vi "Deflate IWT Coeff.vi"(8 "error in (no error)":errorcluster, 11 "IWT coef":T1(array[cluster])) -> (0 "error out":errorcluster, 2 "Length":i32=1051714, 3 "data string":string)   [LabVIEW 2023]
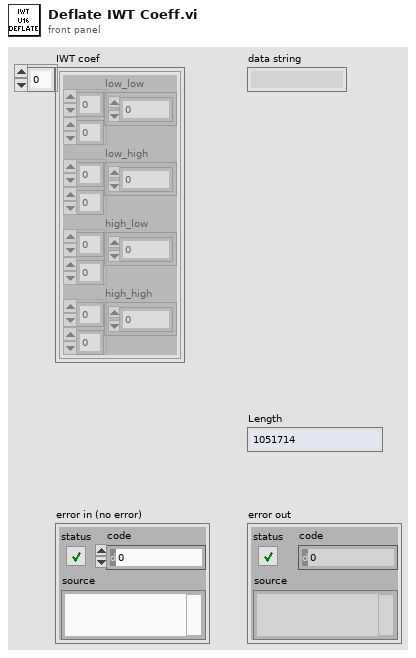
[diagram p1: front panel]
types:
  T1 = cluster{"low_low":i32[][], "low_high":i32[][], "high_low":i32[][], "high_high":i32[][]}[]
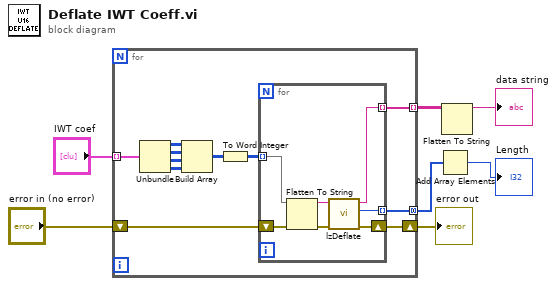
[diagram p0: block diagram]
diagram:
  n1 = for {
    tunnel: "IWT coef" -> [w18] mode=indexing
    tunnel: [w13] -> w2 mode=concatenating
    tunnel: [w10] -> w1 mode=indexing
    shift-right: [w8] -> w7
    shift-left: "error in (no error)" -> [w9]
    n2 = Unbundle(w18) -> ("low_low"=w17:i32[][], "low_high"=w16:i32[][], "high_low"=w15:i32[][], "high_high"=w14:i32[][])
    n3 = Build Array(w17, w16, w15, w14) -> (w12:i32[][][])
    n4 = To Word Integer(number=w12) -> (16bit integer=w11:i16[][][])
    n5 = for {
      tunnel: w11 -> [w24] mode=indexing
      tunnel: [w23] -> w13 mode=indexing
      tunnel: [w22] -> w10 mode=indexing
      shift-right: [w19] -> w8
      shift-left: w9 -> [w21]
      n6 = Flatten To String(anything=w24, error in (no error)=w21) -> (data string=w25:string, error out=w20:errorcluster)  [unwired: 2 in, 1 out]
      n7 = call "lzDeflate.vi"("error in (no error)"=w20, "input"=w25) -> ("error out"=w19:errorcluster, "length"=w23:i32, "deflated output"=w22:string)  [unwired: 3 in]
    }
  }
  "error out" <- w7
  n8 = Add Array Elements(numeric array=w2) -> (sum=→"Length":i32)
  n9 = Flatten To String(anything=w1) -> (data string=→"data string":string)  [unwired: 3 in, 2 out]
